vi "BB_Check_Gyro_Direction.vi"(11 "currentCamera":bool) -> (3 "chgCamera":bool)   [LabVIEW 2012]
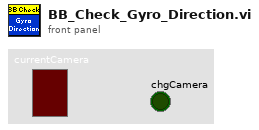
[diagram p1: front panel]
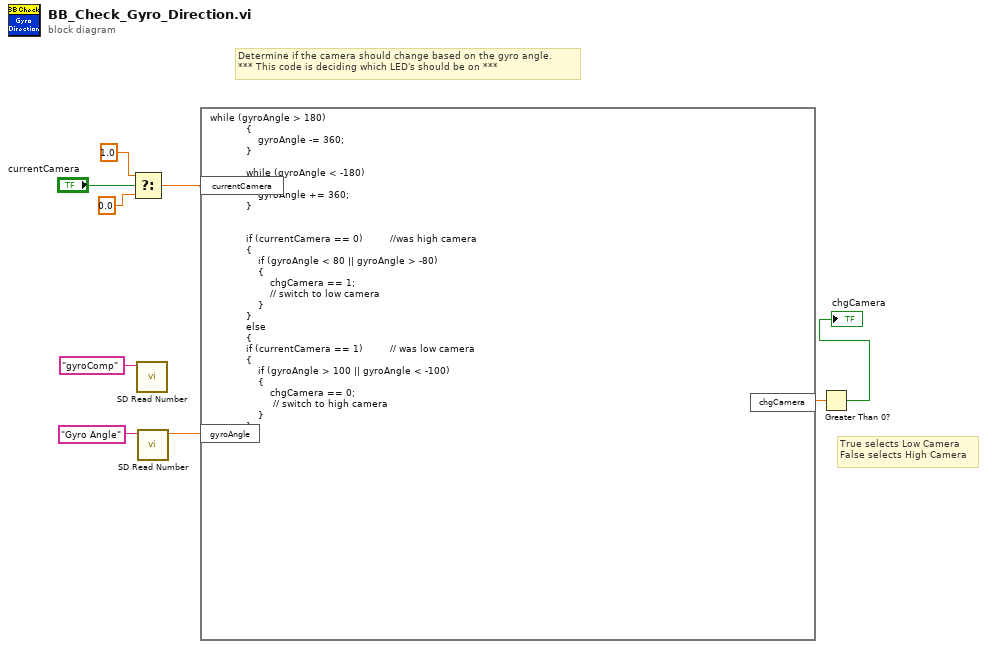
[diagram p0: block diagram]
diagram:
  # "True selects Low Camera\nFalse selects High Camera"
  # "Determine if the camera should change based on the gyro angle.\n*** This code is deciding which LED's should be on ***"
  n1 = Select(t=1.0, s="currentCamera", f=0.0) -> (s? t:f=w1:dbl)
  n2 = call <vilib>:"SD Read Number.vi"("Name"="gyroComp") -> ()  [unwired: 8 in, 3 out]
  n3 = call <vilib>:"SD Read Number.vi"("Name"="Gyro Angle") -> ("Numeric"=w7:dbl)  [unwired: 8 in, 2 out]
  n4 = formula code="while (gyroAngle > 180)\n            {\n                gyroAngle -= 360;  \n            }\n            \n            while (gyroAngle < -180)\n            {\n                gyroAngle += 360;\n            }\n            \n\n            if (currentCamera == 0)         //was high camera\n            {\n                if (gyroAngle < 80 || gyroAngle > -80)\n                {\n                    chgCamera == 1;\n                    // switch to low camera\n                }   \n            }\n            else\n            {\n            if (currentCamera == 1)         // was low camera\n            {\n                if (gyroAngle > 100 || gyroAngle < -100)\n                {\n                    chgCamera == 0;\n                     // switch to high camera\n                }\n            }\n            }"("gyroAngle"=w7, "currentCamera"=w1) -> ("chgCamera"=w6:dbl)
  n5 = Greater Than 0?(x=w6) -> (x > 0?=→"chgCamera":bool)
